vi "setImageNumber.vi"(8 "error in (no error)":errorcluster, 10 "image number":i32, 11 "PixelflySettings in":refnum<class "PixelflySettings.lvclass">) -> (0 "error out":errorcluster, 3 "PixelflySettings out":refnum<class "PixelflySettings.lvclass">)   [LabVIEW 2009, in "Tools.lvlib" / "Settings.lvlib" / "PixelflySettings.lvclass"]
uses:
  PixelflySettings.lvclass
  PixelflySettings.lvclass/PixelflySettings.ctl
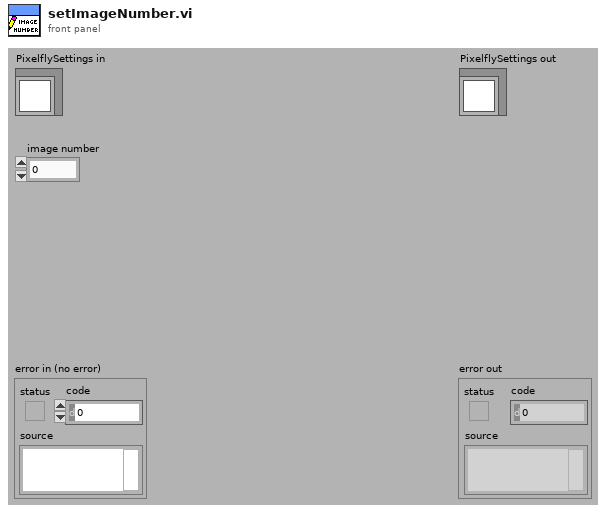
[diagram p1: front panel]
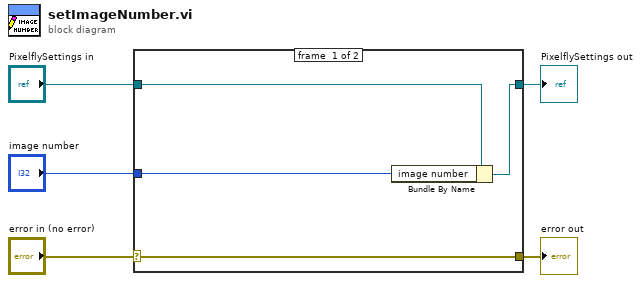
[diagram p0: block diagram]
diagram:
  n1 = case shown="No Error" "error in (no error)" {
    selector: "error in (no error)" -> [w9 w10]
    tunnel: [w9 w10] -> w4
    tunnel: [w7 w11] -> w2
    tunnel: "PixelflySettings in" -> [w8 w11]
    tunnel: "image number" -> [w6 _]
    frame #0 {
      n2 = Bundle By Name(cluster=w8, "image number"=w6) -> (w7:refnum<class "PixelflySettings.lvclass">)
    }
    frame #1 {
    }
  }
  "error out" <- w4
  "PixelflySettings out" <- w2
